vi "FancyPID.vi"(4 "Reset":bool, 6 "Gains":T1={"proportional gain (Kc)"=1.0, "integral time (Ti, min)"=0.01, "derivative time (Td, min)"=0.0} {"derivative time (Td, min)" format="%.3f"; "integral time (Ti, min)" format="%.3f"; "proportional gain (Kc)" format="%.3f"}, 7 "Range":cluster{"output high":dbl, "output low":dbl}={"output high"=0.6, "output low"=-0.6} {"output low" format="%.2f"; "output high" format="%.2f"}, 8 "Disable Range":dbl, 9 "Integral Range":dbl=10000.0, 10 "Process variable":dbl, 11 "Setpoint":dbl) -> (3 "output":dbl format="%.2f")   [LabVIEW 2017]
doc: "PID with integral term only enabled in a range around the setpoint, and the ouput being 0 in a range around the setpoint"
uses:
  <vilib>/addons/control/pid/pid.llb/PID (DBL).vi
  <vilib>/addons/control/pid/NI_PID_pid.lvlib
panel:
  out "Chart":cluster{"Setpoint":dbl, "Process variable":dbl}(graph)
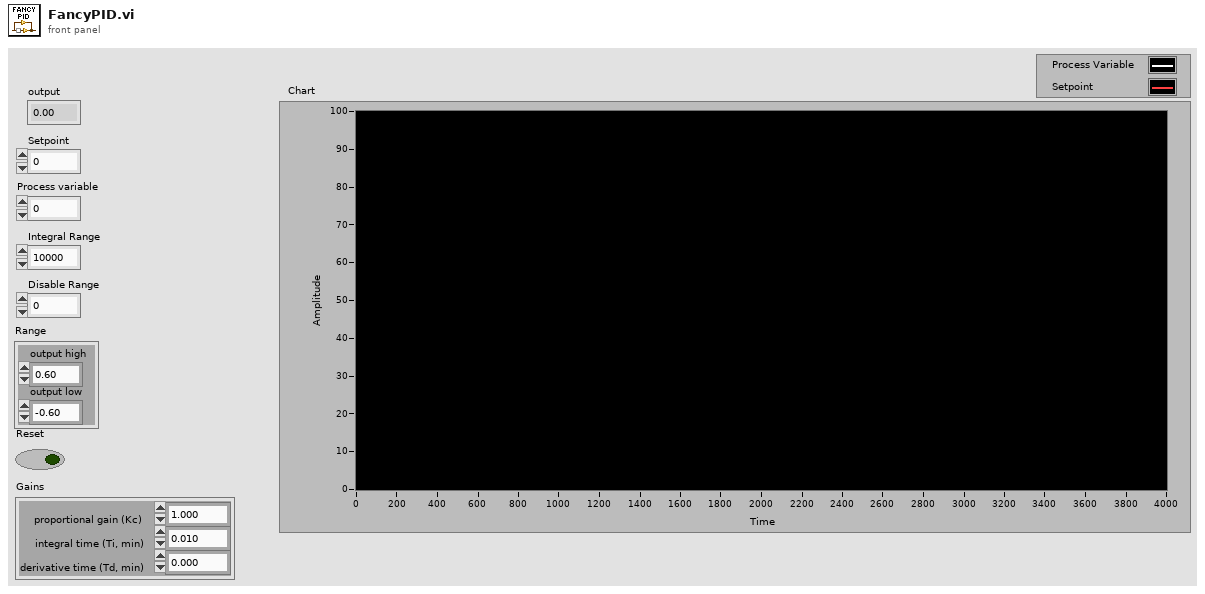
[diagram p1: front panel]
types:
  T1 = cluster{"proportional gain (Kc)":dbl, "integral time (Ti, min)":dbl, "derivative time (Td, min)":dbl}
  T2 = cluster{"proportional gain (Kc)":dbl, "f":dbl, "derivative time (Td, min)":dbl}
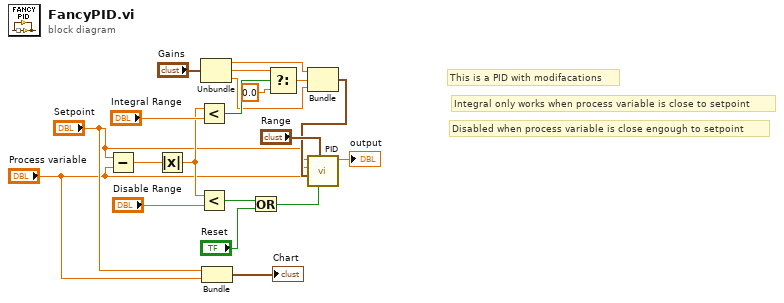
[diagram p0: block diagram]
diagram:
  # "This is a PID with modifacations"
  # "Disabled when process variable is close engough to setpoint"
  # "Integral only works when process variable is close to setpoint"
  n1 = Subtract(x="Setpoint", y="Process variable") -> (x-y=w19:dbl)
  n2 = Absolute Value(x=w19) -> (abs(x)=w9:dbl)
  n3 = Less?(x=w9, y="Integral Range") -> (x < y?=w17:bool)
  n4 = Less?(x=w9, y="Disable Range") -> (x < y?=w7:bool)
  n5 = Unbundle("Gains") -> ("proportional gain (Kc)"=w12:dbl, "integral time (Ti, min)"=w15:dbl, "derivative time (Td, min)"=w11:dbl)
  n6 = Bundle("Setpoint"="Setpoint", "Process variable"="Process variable") -> (→"Chart":cluster{"Setpoint":dbl, "Process variable":dbl})  [unwired: 1 in]
  n7 = Or(x=w7, y="Reset") -> (x .or. y?=w6:bool)
  n8 = Select(t=w15, s=w17, f=0.0) -> (s? t:f=w13:dbl)
  n9 = Bundle("proportional gain (Kc)"=w12, "f"=w13, "derivative time (Td, min)"=w11) -> (w4:T2)  [unwired: 1 in]
  n10 = call-poly <vilib>:"PID.vi"("reinitialize? (F)"=w6, "output range"="Range", "PID gains"=w4, "process variable"="Process variable", "setpoint"="Setpoint") -> ("output"=→"output":dbl)  [unwired: 5 in, 1 out]
